vi "emi_Close VI Reference.vi"(2 "Close ref?(T)":bool=TRUE, 5 "VI Refnum":refnum<vi>, 9 "error in (no error)":errorcluster) -> (6 "VI Refnum Out":refnum<vi>, 10 "error out":errorcluster)   [LabVIEW 2011]
doc: "Close a VI refrence if Close ref?(T) Is True.\nFunction is performed regardless of error in.\n\nIntended for use together with the conditional create VI ref vi's. (Connect \"Ref Created to\"s \"Close ref?\""
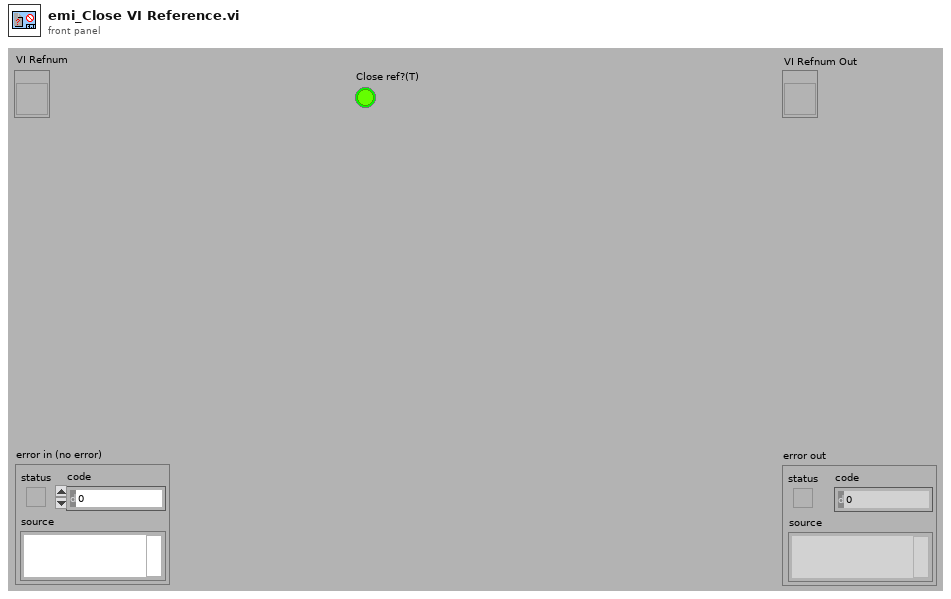
[diagram p1: front panel]
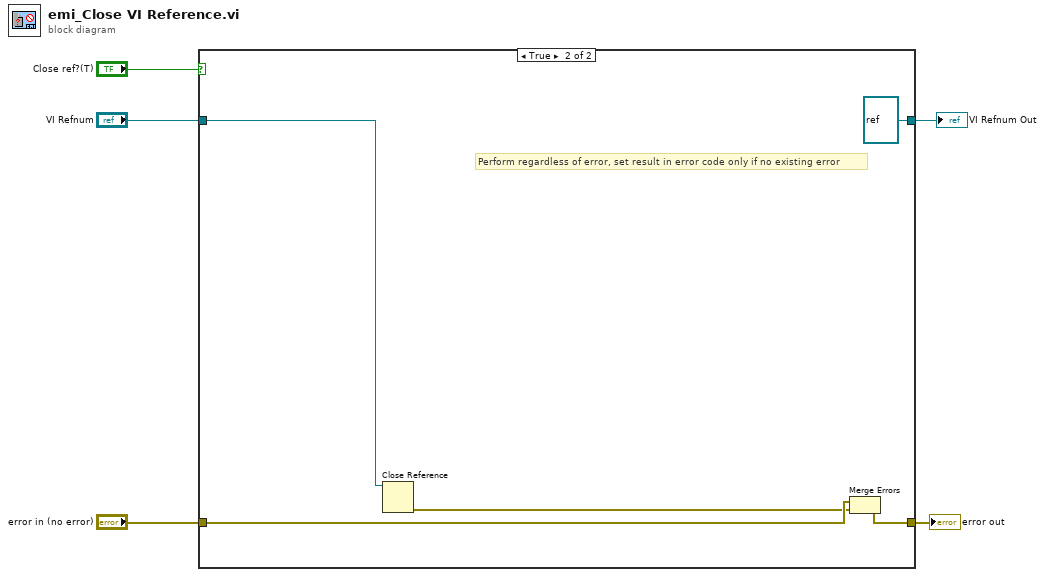
[diagram p0: block diagram]
diagram:
  n1 = case shown="True" "Close ref?(T)" {
    tunnel: [w6 w12] -> w5
    tunnel: [w7 refnum<vi> refnum ("VI Refnum")] -> w4
    tunnel: "VI Refnum" -> [w7 w9]
    tunnel: "error in (no error)" -> [w6 w11]
    frame False {
    }
    frame True {
      # "Perform regardless of error, set result in error code only if no existing error"
      n2 = Close Reference(reference=w9) -> (error out=w10:errorcluster)  [unwired: 1 in]
      n3 = Merge Errors(w11, w10) -> (w12:errorcluster)
    }
  }
  "error out" <- w5
  "VI Refnum Out" <- w4
